vi "Binary Format Investigator.vi"() -> ()   [LabVIEW 2013]
panel:
  out "output array":u8[][](array[numeric])
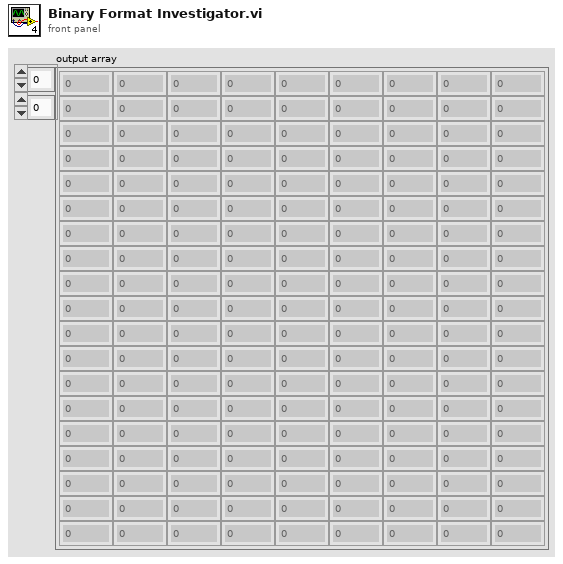
[diagram p1: front panel]
types:
  T1 = enum16{"big-endian, network order", "native, host order", "little-endian"}
  T2 = enum16{"open", "replace", "create", "open or create", "replace or create", "replace or create with confirmation"}
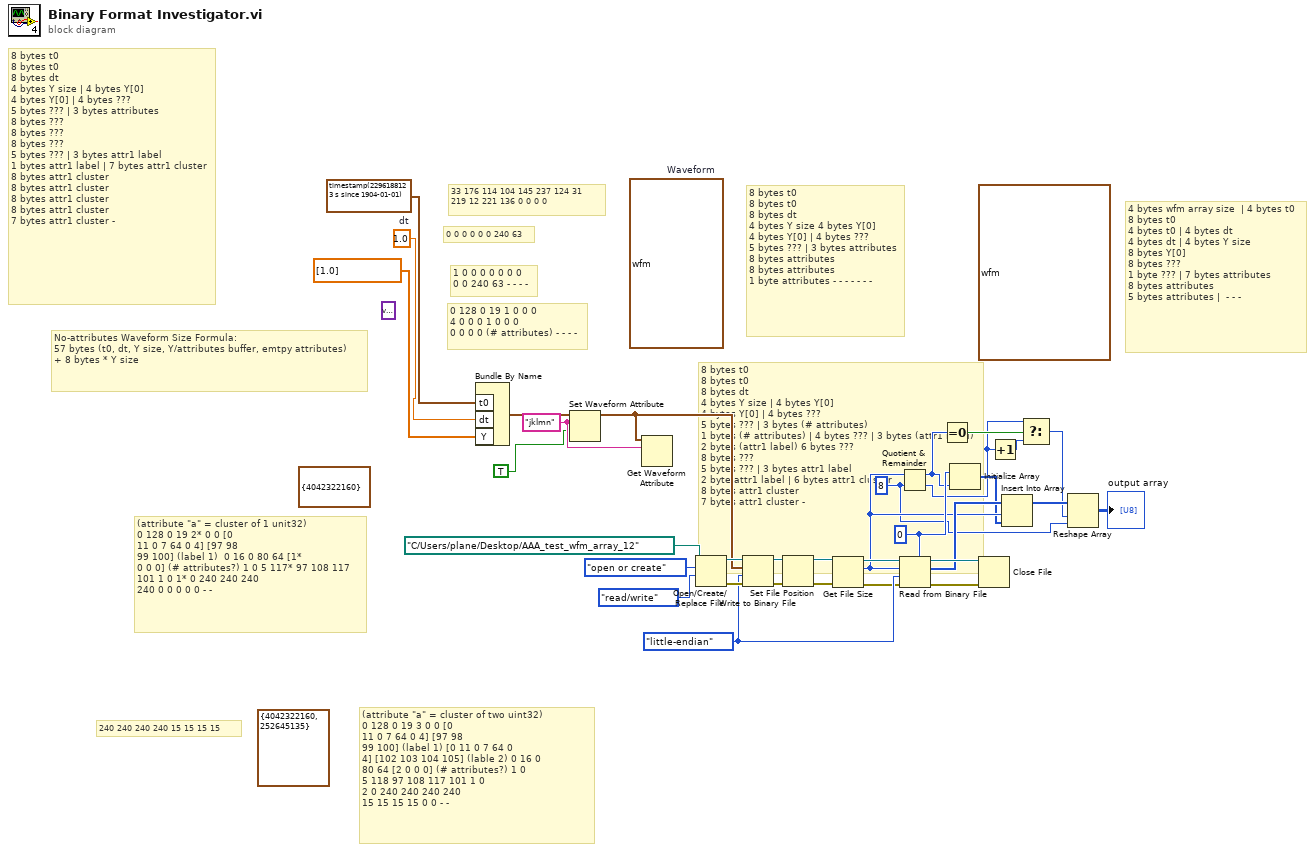
[diagram p0: block diagram]
diagram:
  (unwired) cluster{"abcd":u32, "fghi":u32} {"abcd"=4042322160, "fghi"=252645135} ("value")
  (unwired) cluster{"abcd":u32} {"abcd"=4042322160} ("value")
  w3 = "jklmn" ("name")
  (unwired) waveform(dbl)[] [{"t0"=timestamp(2296188123.123 s since 1904-01-01), "dt"=1.0, "Y"=[1.0]}]
  w10 = i64 8 ("y")
  w20 = u8 0
  (unwired) waveform(dbl) {"t0"=timestamp(2296231323.123 s since 1904-01-01), "dt"=1.0, "Y"=[1.0]}  # Waveform
  (unwired) variant ("attributes")
  w7 = 1.0  # dt
  w27 = T1."little-endian" ("byte order (0:big-endian, network order)")
  # "8 bytes t0\n8 bytes t0\n8 bytes dt\n4 bytes Y size | 4 bytes Y[0]\n4 bytes Y[0] | 4 bytes ???\n5 bytes ??? | 3 bytes attributes\n8 bytes ???\n8 bytes ???\n8 bytes ???\n5 bytes ??? | 3 bytes attr1 label\n1 bytes attr1 label | 7 bytes attr1 cluster\n8 bytes attr1 cluster\n8 bytes attr1 cluster\n8 bytes attr1 cluster\n8 bytes attr1 cluster\n7 bytes attr1 cluster -"
  # "No-attributes Waveform Size Formula:\n57 bytes (t0, dt, Y size, Y/attributes buffer, emtpy attributes)\n+ 8 bytes * Y size"
  # "8 bytes t0\n8 bytes t0\n8 bytes dt\n4 bytes Y size | 4 bytes Y[0]\n4 bytes Y[0] | 4 bytes ???\n5 bytes ??? | 3 bytes (# attributes)\n1 bytes (# attributes) | 4 bytes ??? | 3 bytes (attr1 label)\n2 bytes (attr1 label) 6 bytes ???\n8 bytes ???\n5 bytes ??? | 3 bytes attr1 label\n2 byte attr1 label | 6 bytes attr1 cluster\n8 bytes attr1 cluster\n7 bytes attr1 cluster -"
  # "(attribute \"a\" = cluster of 1 unit32)\n0 128 0 19 2* 0 0 [0\n11 0 7 64 0 4] [97 98\n99 100] (label 1)  0 16 0 80 64 [1*\n0 0 0] (# attributes?) 1 0 5 117* 97 108 117\n101 1 0 1* 0 240 240 240\n240 0 0 0 0 0 - -"
  # "(attribute \"a\" = cluster of two uint32)\n0 128 0 19 3 0 0 [0\n11 0 7 64 0 4] [97 98\n99 100] (label 1) [0 11 0 7 64 0\n4] [102 103 104 105] (lable 2) 0 16 0\n80 64 [2 0 0 0] (# attributes?) 1 0\n5 118 97 108 117 101 1 0\n2 0 240 240 240 240\n15 15 15 15 0 0 - -"
  # "240 240 240 240 15 15 15 15"
  # "4 bytes wfm array size  | 4 bytes t0\n8 bytes t0\n4 bytes t0 | 4 bytes dt\n4 bytes dt | 4 bytes Y size\n8 bytes Y[0]\n8 bytes ???\n1 byte ??? | 7 bytes attributes\n8 bytes attributes\n5 bytes attributes |  - - -"
  # "8 bytes t0\n8 bytes t0\n8 bytes dt\n4 bytes Y size 4 bytes Y[0]\n4 bytes Y[0] | 4 bytes ???\n5 bytes ??? | 3 bytes attributes\n8 bytes attributes\n8 bytes attributes\n1 byte attributes - - - - - - -"
  # "0 128 0 19 1 0 0 0\n4 0 0 0 1 0 0 0\n0 0 0 0 (# attributes) - - - -"
  # "1 0 0 0 0 0 0 0\n0 0 240 63 - - - -"
  # "33 176 114 104 145 237 124 31\n219 12 221 136 0 0 0 0"
  # "0 0 0 0 0 0 240 63"
  n1 = Bundle By Name("t0"=timestamp(2296188123.123 s since 1904-01-01), "dt"=w7, "Y"=dbl[] [1.0]) -> (w4:waveform(dbl))  [unwired: 1 in]
  n2 = Set Waveform Attribute(5:TRUE, 6:w3, 7:w4) -> (3:w2:waveform(dbl))  [unwired: 1 in, 2 out]
  n3 = Get Waveform Attribute(6:w3, 7:w2) -> ()  [unwired: 2 in, 4 out]
  n4 = Open/Create/Replace File(file path (use dialog)=path "C:/Users/plane/Desktop/AAA_test_wfm_array_12", operation (0:open)=T2."open or create", access (0:read/write)=enum16{"read/write", "read-only", "write-only"}."read/write") -> (refnum out=w30:refnum<file>, error out=w31:errorcluster)  [unwired: 3 in, 1 out]
  n5 = Write to Binary File(file (use dialog)=w30, data=w2, error in=w31, 9:w27) -> (refnum out=w26:refnum<file>, error out=w25:errorcluster)  [unwired: 2 in, 1 out]
  n6 = Set File Position(refnum=w26, error in=w25) -> (refnum out=w24:refnum<file>, error out=w23:errorcluster)  [unwired: 2 in]
  n7 = Get File Size(file=w24, error in=w23) -> (refnum out=w22:refnum<file>, size (in bytes)=w18:i64, 0:w21:errorcluster)
  n8 = Quotient & Remainder(x=w18, y=w10) -> (x-y*floor(x/y)=w14:i64, floor(x/y)=w12:i64)
  n9 = Read from Binary File(5:w20, 8:w21, 9:w27, 10:w18, 11:w22) -> (0:w29:errorcluster, 2:w19:u8[], 3:w28:refnum<file>)  [unwired: 1 in, 1 out]
  n10 = Equal To 0?(x=w14) -> (x = 0?=w15:bool)
  n11 = Initialize Array(w20, w14) -> (w17:u8[])
  n12 = Close File(refnum=w28, error in=w29) -> ()  [unwired: 2 out]
  n13 = Increment(x=w12) -> (x+1=w13:i64)
  n14 = Insert Into Array(array=w19, index=w18, new element=w17) -> (w16:u8[])
  n15 = Select(t=w12, s=w15, f=w13) -> (s? t:f=w11:i64)
  n16 = Reshape Array(w16, w11, w10) -> (→"output array":u8[][])
